vi "set_value.vi"(8 "error in (no error)":errorcluster, 10 "value":string, 11 "self in":refnum<class "Identifier.lvclass">) -> (0 "error out":errorcluster, 3 "self out":refnum<class "Identifier.lvclass">)   [LabVIEW 2020, in "mlir.lvlib" / "Identifier.lvclass"]
uses:
  Identifier.lvclass
  Identifier.lvclass/Identifier.ctl
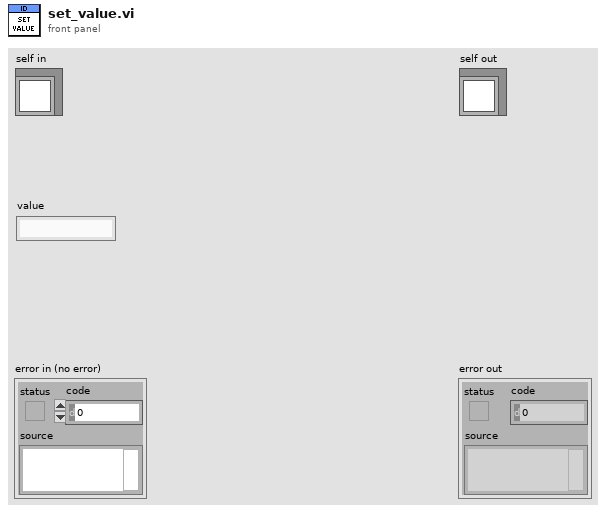
[diagram p1: front panel]
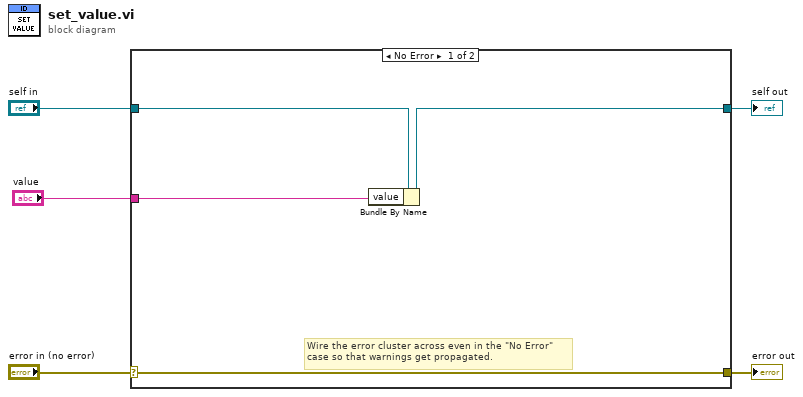
[diagram p0: block diagram]
diagram:
  n1 = case shown="No Error" "error in (no error)" {
    selector: "error in (no error)" -> [w8 w11]
    tunnel: [w8 w11] -> w4
    tunnel: [w7 w10] -> w2
    tunnel: "self in" -> [w9 w10]
    tunnel: "value" -> [w6 _]
    frame No Error {
      # "Wire the error cluster across even in the \"No Error\"\ncase so that warnings get propagated."
      n2 = Bundle By Name(cluster=w9, "value"=w6) -> (w7:refnum<class "Identifier.lvclass">)
    }
    frame Error {
    }
  }
  "error out" <- w4
  "self out" <- w2
